vi "ObtainAppInfo.vi"(7 "Set (f)":bool, 11 "testAppRefs":T1={"RingdownConfig"=refnum, "AppType"="none"}) -> (3 "testAppRefs":T1)   [LabVIEW 2014, in "AppModule.lvlib"]
uses:
  AppModule.lvlib
  Test/TestAppRefs.ctl
  AppPlugins/RingdownPlugin/PublicAPI/TypeDef/RingdownConfig.ctl
  AppPlugins/RingdownPlugin/RingdownPlugin.lvclass
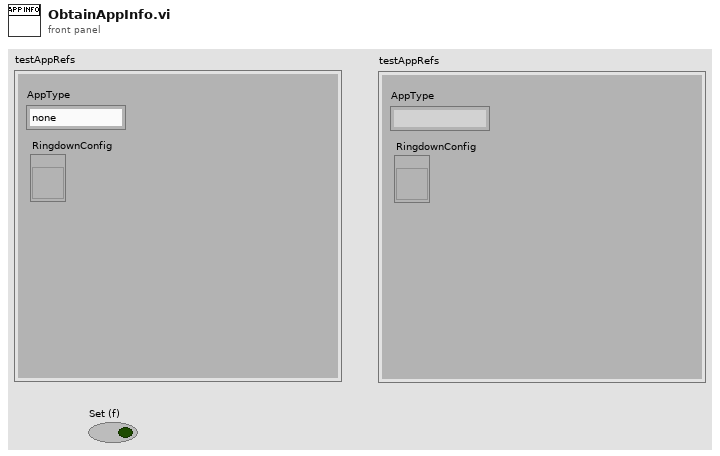
[diagram p1: front panel]
types:
  T1 = typedef "AppModule.lvlib/TestAppRefs.ctl" = cluster{"RingdownConfig":refnum<vi>, "AppType":string}
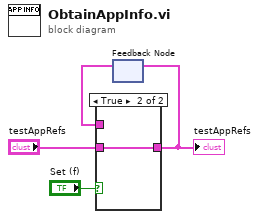
[diagram p0: block diagram]
diagram:
  n1 = feedback #1() -> (w1:T1)  [unwired: 1 in]
  n2 = case shown="True" "Set (f)" {
    tunnel: "testAppRefs" -> [_ w6]
    tunnel: [w5 w6] -> w3
    tunnel: w1 -> [w5 _]
    frame False {
    }
    frame True {
    }
  }
  "testAppRefs" <- w3
  n3 = feedback-in #1(w3) -> ()
